vi "OnButtonArray.vi"(0 "Input":bool[](array[boolean])) -> (1 "Pressed":bool[](array[boolean]), 2 "Released":bool[](array[boolean]))   [LabVIEW 2016]
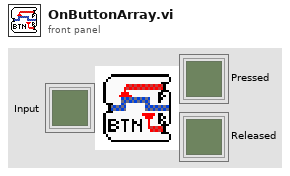
[diagram p1: front panel]
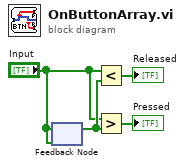
[diagram p0: block diagram]
diagram:
  n1 = feedback-in #1("Input") -> ()
  n2 = feedback #1("Input") -> (w4:bool[])
  n3 = Less?(x="Input", y=w4) -> (x < y?=→"Released":bool[])
  n4 = Greater?(x="Input", y=w4) -> (0:→"Pressed":bool[])
